vi "uc480_SimpleLive.vi"() -> ()   [LabVIEW 2018]
uses:
  System.Windows.Forms
  C:/Program Files/National Instruments/LabVIEW 2018/uc480DotNet.dll
  Program Files/National Instruments/LabVIEW 2018/uc480DotNet.dll
panel:
  in  "Zoom":u16(ring)=1 items=["4X"=4, "2X"=2, "1X"=1]
  in  "PictureBox":refnum<k24>(container)
  out "Serial Number 2":string
  out "Height 2":i32=8
  out "Width 2":i32=8
  out "Bits/Pixel 2":i32=8
  in  "Camera ID":i32
  out "Serial Number":string
  out "Height":i32=8
  out "Width":i32=8
  out "Bits/Pixel":i32=8
  in  "Pixelclock":i32(slide)=33 min=5 max=30 step=1 scale=5.0..30.0
  in  "Framerate":dbl(slide)=33.21525 min=2.938631097475863 max=10.003070942779434 step=0.008308198457458001 scale=2.938631097475863..10.003070942779434 scale format="%#.3g"
  in  "Exposure":dbl(slide)=33.21525 min=0.11904999999999999 max=99.92214999999999 step=0.0831 scale=0.11904999999999999..99.92214999999999 scale format="%#.3g"
  out "Error Out":errorcluster caption="error"
  in  "Load Parameter":bool
  in  "Exit Camera":bool
  in  "Stop Live":bool
  in  "Start Live":bool
  in  "Init Camera":bool
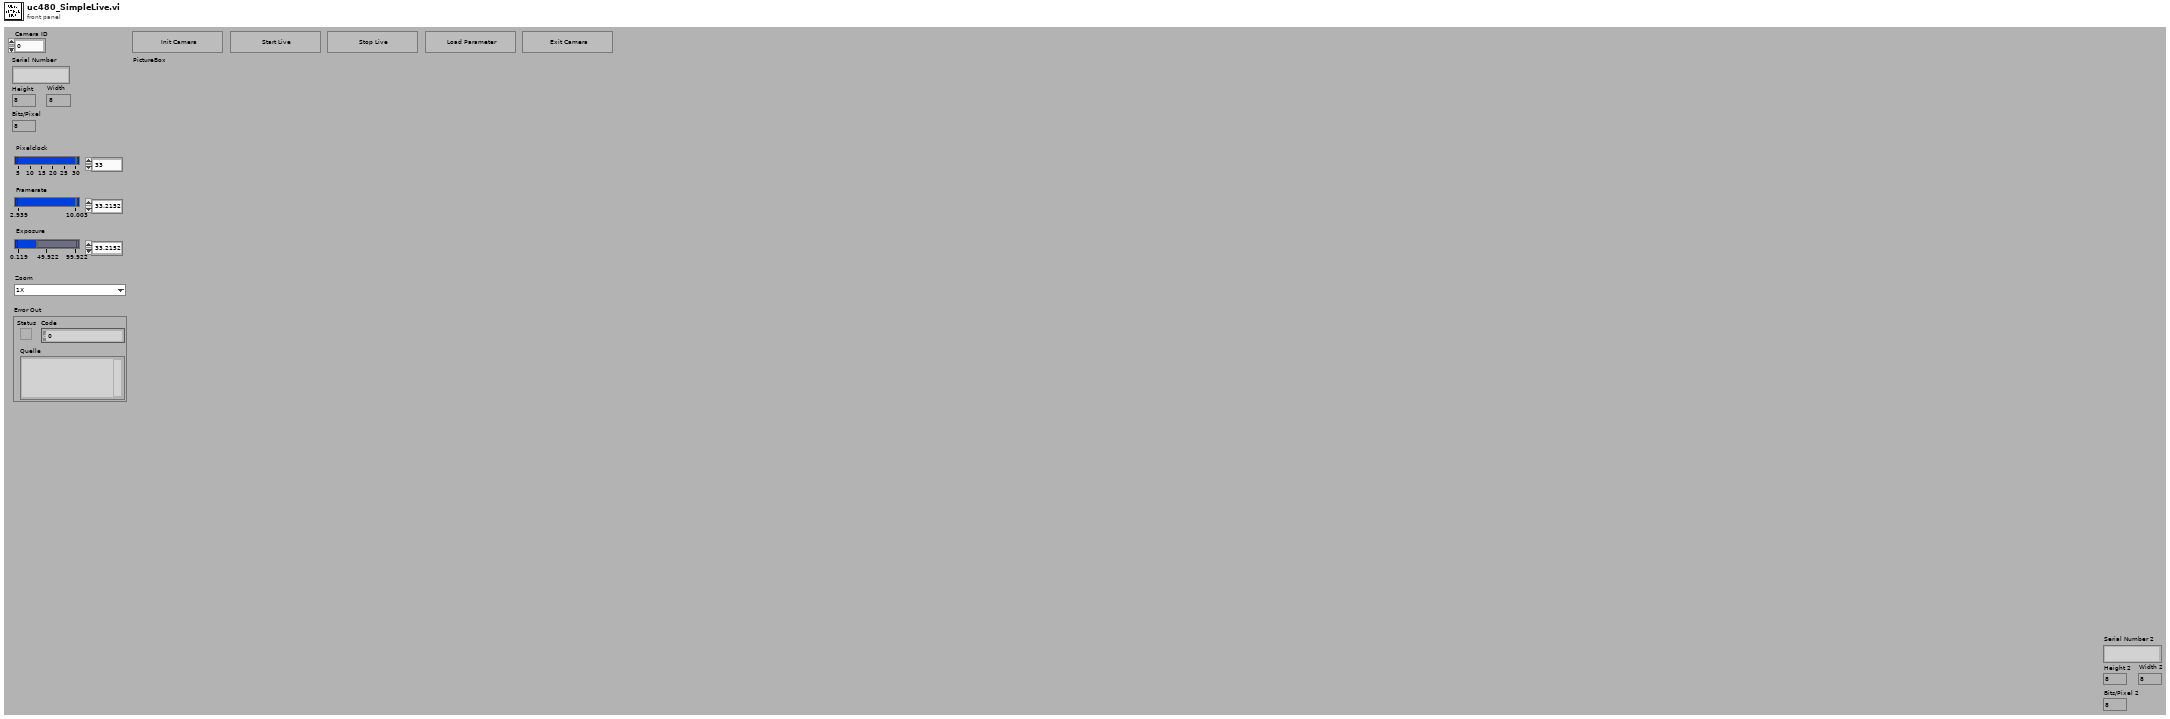
[diagram p1: front panel]
types:
  T1 = enum8{"Enabled", "Disabled", "Disabled and Grayed Out"}
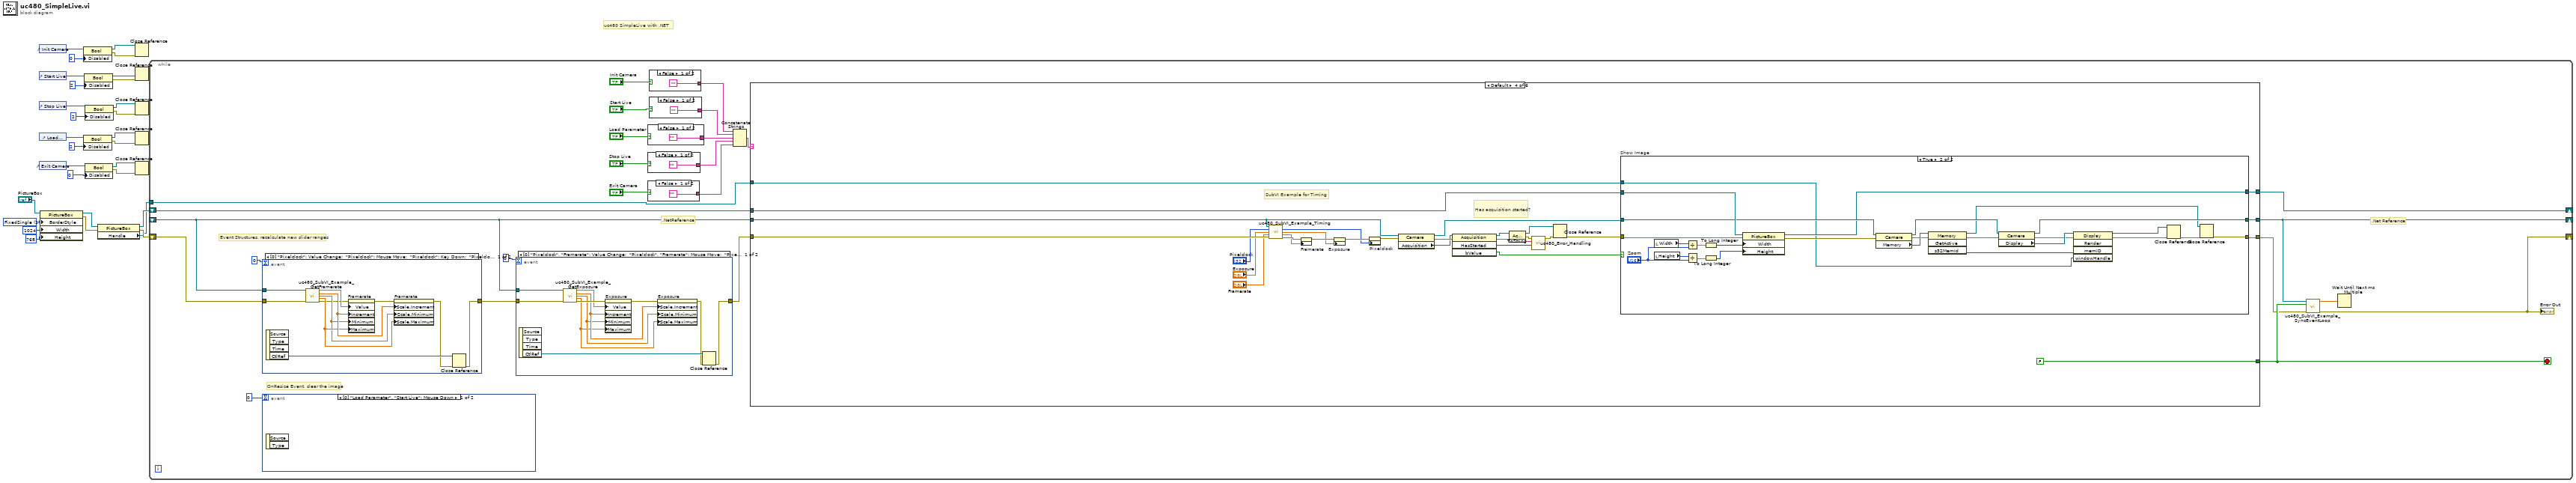
[diagram p0: block diagram]
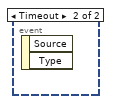
[diagram p2: hidden frame]
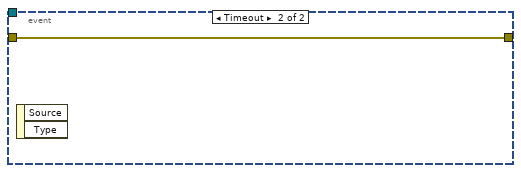
[diagram p3: hidden frame]
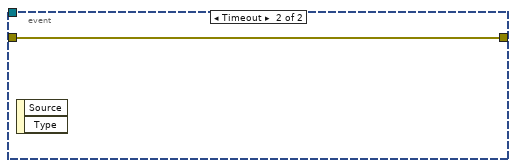
[diagram p4: hidden frame]
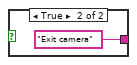
[diagram p5: hidden frame]
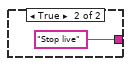
[diagram p6: hidden frame]
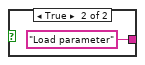
[diagram p7: hidden frame]
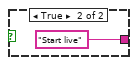
[diagram p8: hidden frame]
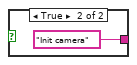
[diagram p9: hidden frame]
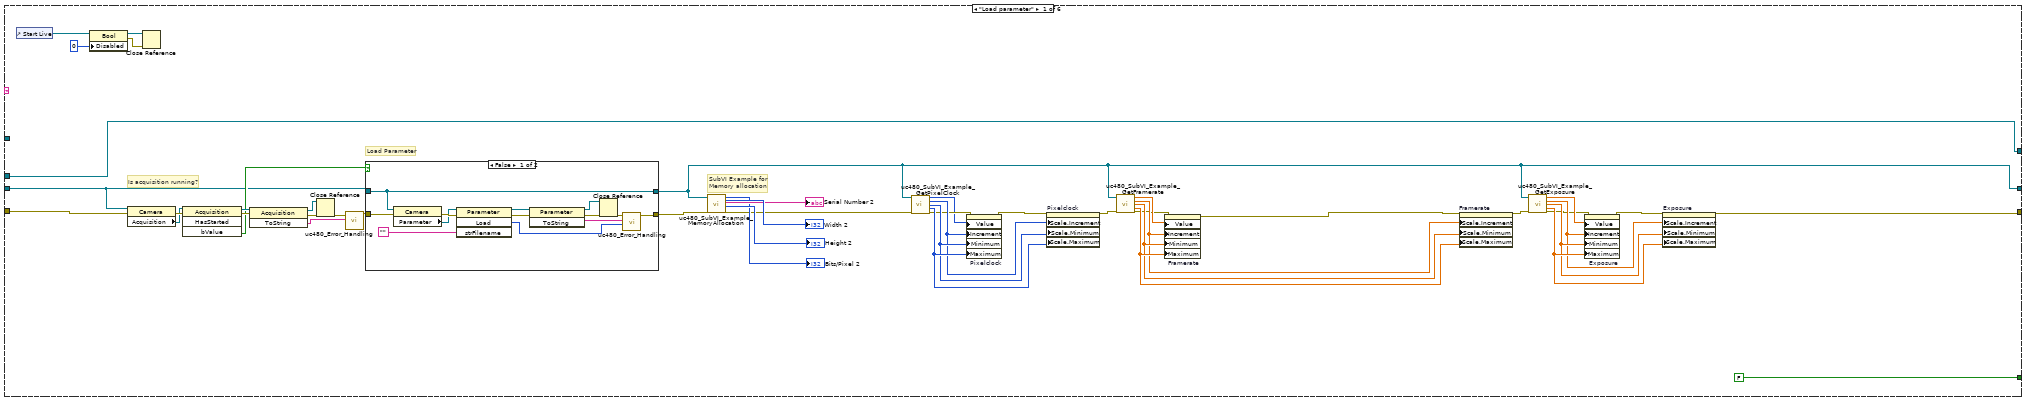
[diagram p10: hidden frame]
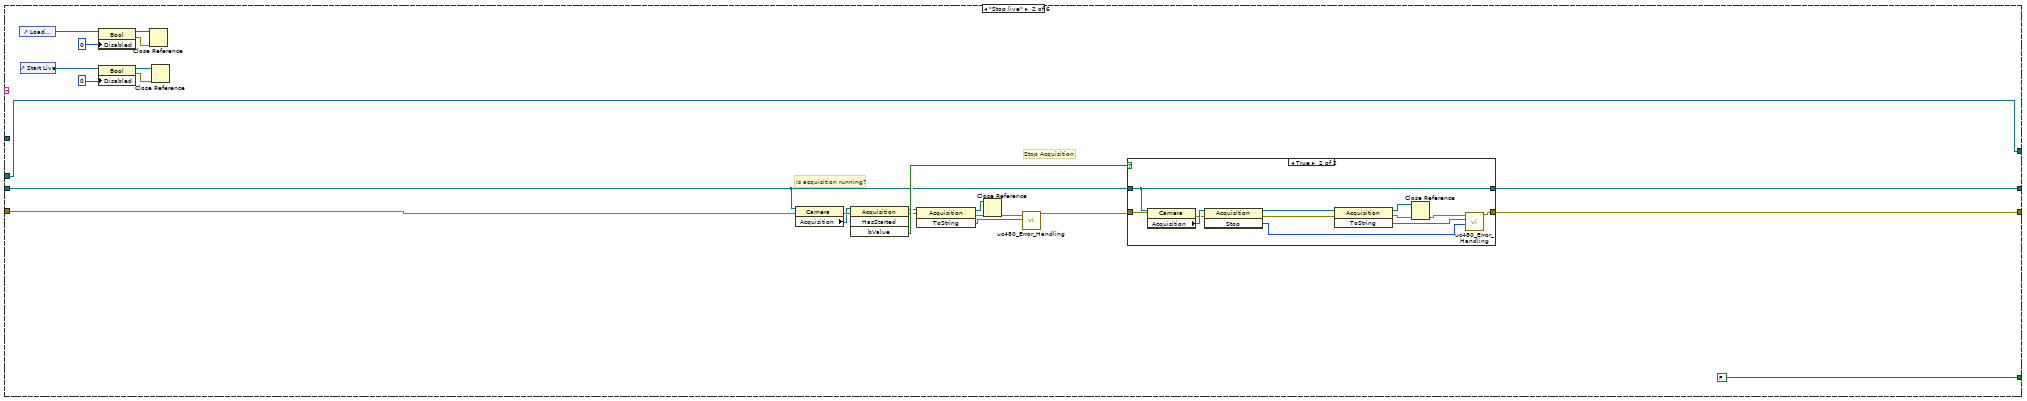
[diagram p12: hidden frame]
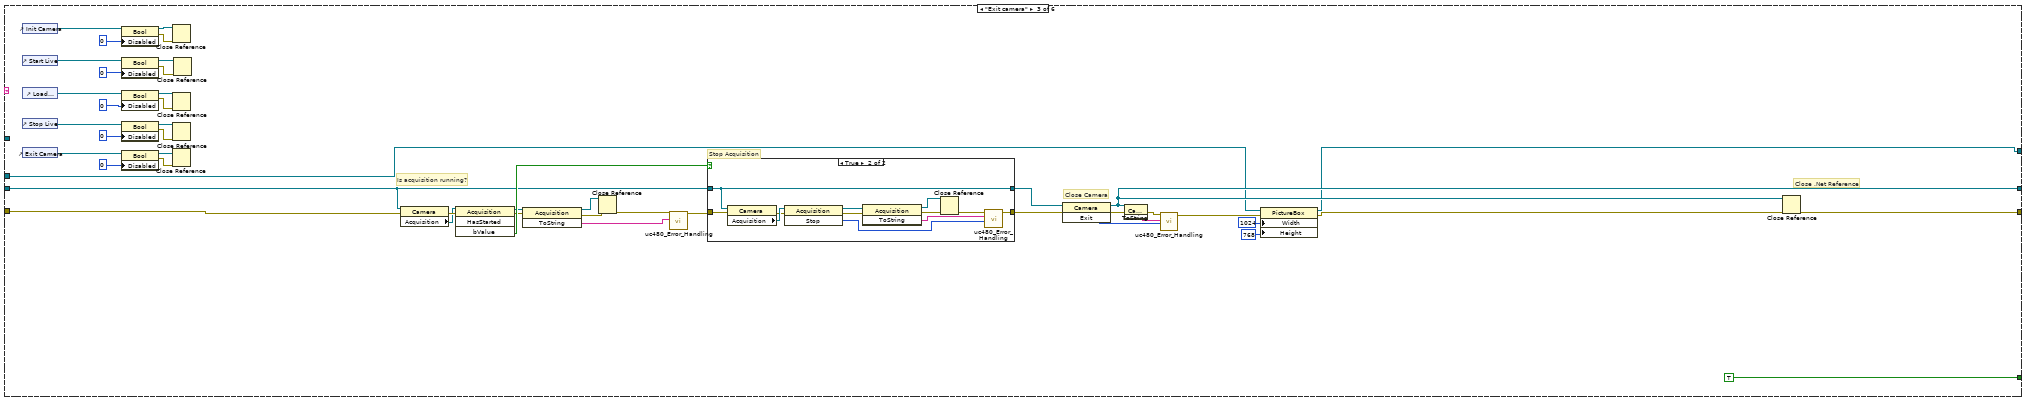
[diagram p14: hidden frame]
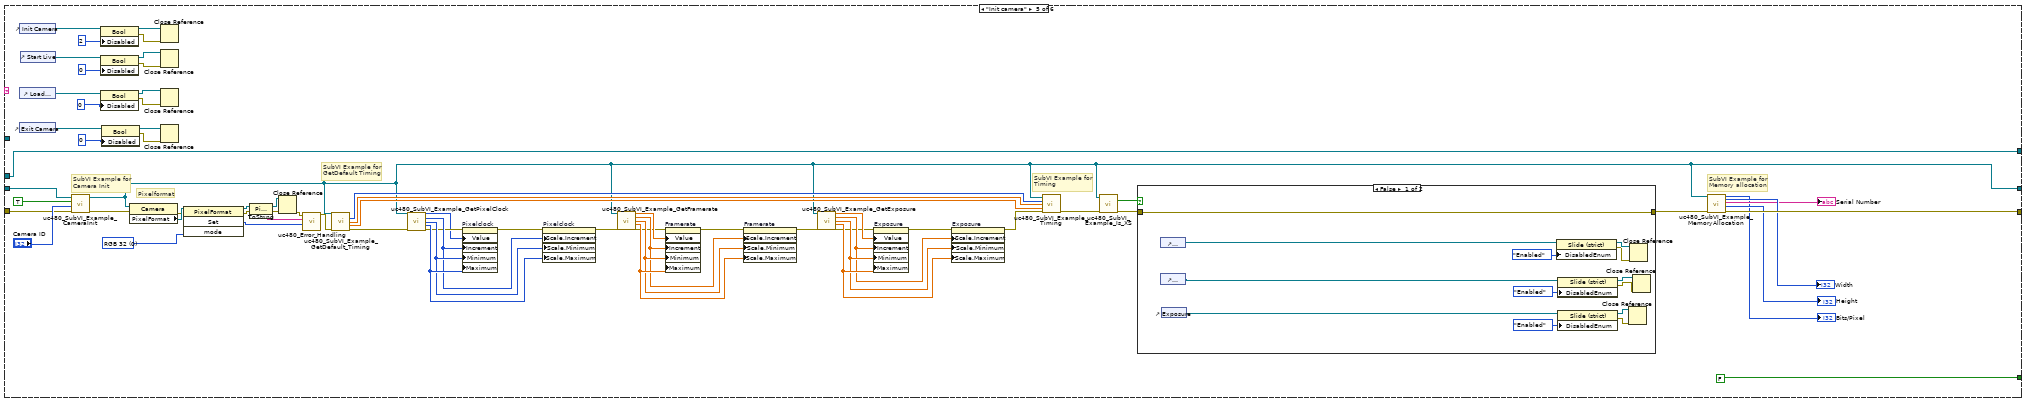
[diagram p17: hidden frame]
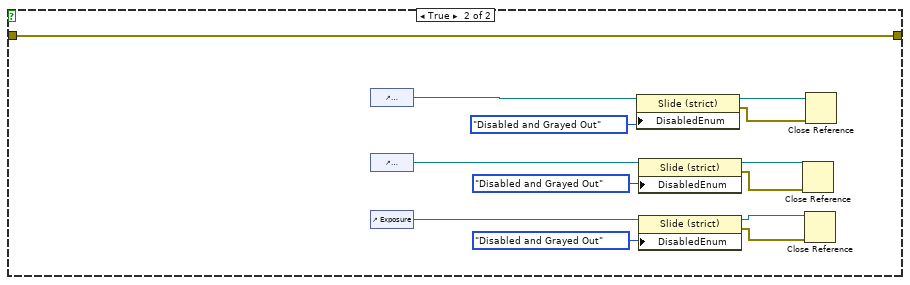
[diagram p18: hidden frame]
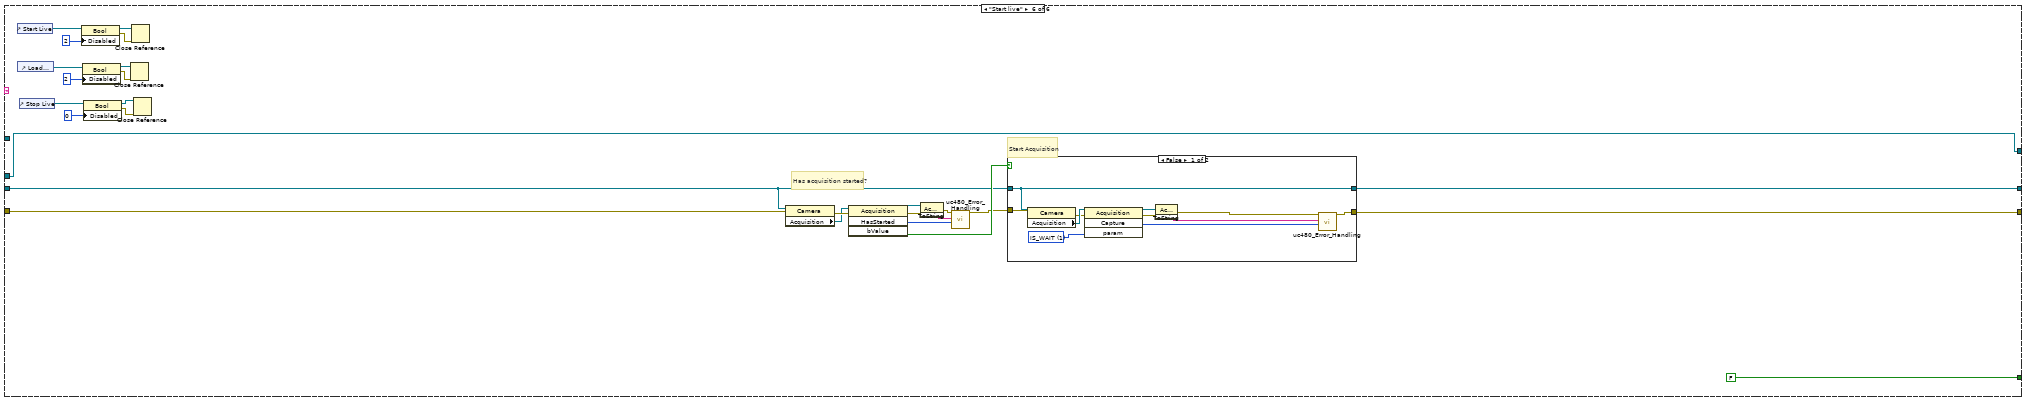
[diagram p19: hidden frame]
diagram:
  w18 = 1 items=["None", "FixedSingle", "Fixed3D"] ("BorderStyle")
  # "uc480 SimpleLive with .NET"
  n1 = control-ref of="Init Camera"() -> (w29:refnum<vi>)
  n2 = control-ref of="Start Live"() -> (w26:refnum<vi>)
  n3 = control-ref of="Stop Live"() -> (w20:refnum<vi>)
  n4 = control-ref of="Load Parameter"() -> (w21:refnum<vi>)
  n5 = control-ref of="Exit Camera"() -> (w22:refnum<vi>)
  n6 = property class="PictureBox"(reference="PictureBox", "BorderStyle"=w18, "Width"=1024, "Height"=768) -> (reference out=w4:refnum<k24>, error out=w5:errorcluster)  [unwired: 1 in]
  n7 = property class="Bool"(reference=w29, "Disabled"=u8 0 ("Deaktiviert")) -> (reference out=w15:refnum<vi>, error out=w14:errorcluster)  [unwired: 1 in]
  n8 = property class="Bool"(reference=w21, "Disabled"=u8 2 ("Deaktiviert")) -> (reference out=w9:refnum<vi>, error out=w8:errorcluster)  [unwired: 1 in]
  n9 = property class="Bool"(reference=w26, "Disabled"=u8 2 ("Deaktiviert")) -> (reference out=w13:refnum<vi>, error out=w12:errorcluster)  [unwired: 1 in]
  n10 = property class="Bool"(reference=w22, "Disabled"=u8 0 ("Deaktiviert")) -> (reference out=w7:refnum<vi>, error out=w6:errorcluster)  [unwired: 1 in]
  n11 = property class="Bool"(reference=w20, "Disabled"=u8 2 ("Deaktiviert")) -> (reference out=w11:refnum<vi>, error out=w10:errorcluster)  [unwired: 1 in]
  n12 = property class="PictureBox"(reference=w4, error in=w5) -> (reference out=w3:refnum<k24>, error out=w2:errorcluster, "Handle"=w1:refnum<k24>)
  n13 = Close Reference(reference=w15, error in (no error)=w14) -> ()  [unwired: 1 out]
  n14 = Close Reference(reference=w13, error in (no error)=w12) -> ()  [unwired: 1 out]
  n15 = Close Reference(reference=w11, error in (no error)=w10) -> ()  [unwired: 1 out]
  n16 = Close Reference(reference=w9, error in (no error)=w8) -> ()  [unwired: 1 out]
  n17 = Close Reference(reference=w7, error in (no error)=w6) -> ()  [unwired: 1 out]
  n18 = while {
    shift-right: [w34] -> _
    shift-left: w2 -> [w40]
    shift-right: [w37] -> _
    shift-left: _ -> [w30]
    shift-right: [w32] -> _
    shift-left: w3 -> [w33]
    tunnel: w1 -> [w31]
    stop <- w38 stop-if-true
    # "OnResize Event, clear the image"
    # "Event Structures, recalculate new slider ranges"
    # ".NetReference"
    # ".Net Reference"
    n19 = event shown="[0] \"Pixelclock\": Value Change;  \"Pixelclock\": Mouse Move;  \"Pixelclock\": Key Down;  \"Pixelclock\": Mouse Up" {
      selector: _ -> [_ _]
      dyn-events: _ -> [_ _]
      timeout: 0 -> [_ _]
      tunnel: [w56 w67] -> w41
      tunnel: w40 -> [w66 w67]
      tunnel: w30 -> [w65 _]
      event "Pixelclock": Value Change; "Pixelclock": Mouse Move; "Pixelclock": Key Down; "Pixelclock": Mouse Up {
        n20 = event-data() -> ("CtlRef"=w58:refnum<vi>)  [unwired: 1 in, 3 out]
        n21 = call "uc480_SubVI_Example_GetFramerate.vi"(".NET (Reference)"=w65, "Error In"=w66) -> ("Framerate"=w64:dbl, "Inc"=w63:dbl, "Min"=w61:dbl, "Max"=w62:dbl, "error out"=w60:errorcluster)  [unwired: 9 in]
        n22 = property on="Framerate" class="Slide (strict)"(error in=w60, "Value"=w64, "Increment"=w63, "Minimum"=w61, "Maximum"=w62) -> (error out=w59:errorcluster)  [unwired: 1 in, 1 out]
        n23 = property on="Framerate" class="Slide (strict)"(error in=w59, "Scale.Increment"=w63, "Scale.Minimum"=w61, "Scale.Maximum"=w62) -> (error out=w57:errorcluster)  [unwired: 1 in, 1 out]
        n24 = Close Reference(reference=w58, error in (no error)=w57) -> (error out=w56:errorcluster)
      }
      event Timeout {
        n25 = event-data() -> ()  [unwired: 1 in, 2 out]
      }
    }
    n26 = event shown="[0] \"Load Parameter\", \"Start Live\": Mouse Down" {
      selector: _ -> [_ _]
      dyn-events: _ -> [_ _]
      timeout: 0 -> [_ _]
      event "Load Parameter", "Start Live": Mouse Down {
        n27 = event-data() -> ()  [unwired: 1 in, 2 out]
      }
      event Timeout {
        n28 = event-data() -> ()  [unwired: 1 in, 2 out]
      }
    }
    n29 = event shown="[0] \"Pixelclock\", \"Framerate\": Value Change;  \"Pixelclock\", \"Framerate\": Mouse Move;  \"Pixelclock\", \"Framerate\": Key Down;  \"Pixelclock\", \"Framerate\": Mouse Up" {
      selector: _ -> [_ _]
      dyn-events: _ -> [_ _]
      timeout: 0 -> [_ _]
      tunnel: w41 -> [w78 w79]
      tunnel: [w68 w79] -> w43
      tunnel: w30 -> [w77 _]
      event "Pixelclock", "Framerate": Value Change; "Pixelclock", "Framerate": Mouse Move; "Pixelclock", "Framerate": Key Down; "Pixelclock", "Framerate": Mouse Up {
        n30 = event-data() -> ("CtlRef"=w70:refnum<vi>)  [unwired: 1 in, 3 out]
        n31 = call "uc480_SubVI_Example_GetExposure.vi"(".NET (Reference)"=w77, "Error In"=w78) -> ("Exposure"=w74:dbl, "Inc"=w73:dbl, "Min"=w72:dbl, "Max"=w71:dbl, "Error out"=w75:errorcluster)  [unwired: 9 in]
        n32 = property on="Exposure" class="Slide (strict)"(error in=w75, "Value"=w74, "Increment"=w73, "Minimum"=w72, "Maximum"=w71) -> (error out=w76:errorcluster)  [unwired: 1 in, 1 out]
        n33 = property on="Exposure" class="Slide (strict)"(error in=w76, "Scale.Increment"=w73, "Scale.Minimum"=w72, "Scale.Maximum"=w71) -> (error out=w69:errorcluster)  [unwired: 1 in, 1 out]
        n34 = Close Reference(reference=w70, error in (no error)=w69) -> (error out=w68:errorcluster)
      }
      event Timeout {
        n35 = event-data() -> ()  [unwired: 1 in, 2 out]
      }
    }
    n36 = case shown="False" "Exit Camera" {
      tunnel: ["" "Exit camera"] -> w45
      frame False {
      }
      frame True {
      }
    }
    n37 = case shown="False" "Load Parameter" {
      tunnel: ["" "Load parameter"] -> w49
      frame False {
      }
      frame True {
      }
    }
    n38 = case shown="False" "Stop Live" {
      tunnel: ["" "Stop live"] -> w48
      frame False {
      }
      frame True {
      }
    }
    n39 = case shown="False" "Init Camera" {
      tunnel: ["" "Init camera"] -> w53
      frame False {
      }
      frame True {
      }
    }
    n40 = case shown="False" "Start Live" {
      tunnel: ["" "Start live"] -> w52
      frame False {
      }
      frame True {
      }
    }
    n41 = Concatenate Strings(w53, w52, w49, w48, w45) -> (w51:string)
    n42 = case shown="Default" w51 {
      tunnel: w30 -> [w126 w166 w220 w262 w369 w420]
      tunnel: w43 -> [w129 w167 w221 w272 w368 w421]
      tunnel: [w96 w165 w229 w271 w325 w419] -> w37
      tunnel: [w97 w164 w230 w270 w364 w417] -> w36
      tunnel: [FALSE FALSE TRUE FALSE FALSE FALSE] -> w38
      tunnel: w33 -> [w95 w158 w200 w254 w320 w410]
      tunnel: [w95 w158 w199 w253 w320 w410] -> w32
      tunnel: w31 -> [_ _ _ w250 _ _]
      frame "Load parameter" {
        # "SubVI Example for \nMemory allocation"
        # "Is acquisition running?"
        # "Load Parameter"
        n43 = control-ref of="Start Live"() -> (w120:refnum<vi>)
        n44 = property class="Bool"(reference=w120, "Disabled"=u8 0 ("Deaktiviert")) -> (reference out=w94:refnum<vi>, error out=w93:errorcluster)  [unwired: 1 in]
        n45 = property class="Camera"(reference=w126, error in=w129) -> (error out=w134:errorcluster, "Acquisition"=w133:refnum<k24>)  [unwired: 1 out]
        n46 = Close Reference(reference=w94, error in (no error)=w93) -> ()  [unwired: 1 out]
        n47 = invoke class="Acquisition" method="HasStarted"(reference=w133, error in=w134) -> (reference out=w130:refnum<k24>, error out=w132:errorcluster, "bValue"=w128:bool)  [unwired: 2 in, 1 out]
        n48 = invoke class="Acquisition" method="ToString"(reference=w130, error in=w132) -> (reference out=w92:refnum<k24>, error out=w91:errorcluster, "ToString"=w131:string)  [unwired: 1 in]
        n49 = Close Reference(reference=w92, error in (no error)=w91) -> (error out=w90:errorcluster)
        n50 = call "uc480_Error_Handling.vi"("Error String"=w131, "Error In"=w90) -> ("Error Out"=w127:errorcluster)  [unwired: 9 in]
        n51 = case shown="False" w128 {
          tunnel: w127 -> [w142 w149]
          tunnel: w126 -> [w140 w150]
          tunnel: [w141 w149] -> w121
          tunnel: [w140 w150] -> w96
          frame False {
            n52 = property class="Camera"(reference=w140, error in=w142) -> (error out=w144:errorcluster, "Parameter"=w143:refnum<k24>)  [unwired: 1 out]
            n53 = invoke class="Parameter" method="Load"(reference=w143, error in=w144, "strFilename"="") -> (reference out=w146:refnum<k24>, error out=w147:errorcluster, "Load"=w139:i32)  [unwired: 1 in, 1 out]
            n54 = invoke class="Parameter" method="ToString"(reference=w146, error in=w147) -> (reference out=w136:refnum<k24>, error out=w138:errorcluster, "ToString"=w148:string)  [unwired: 1 in]
            n55 = Close Reference(reference=w136, error in (no error)=w138) -> (error out=w137:errorcluster)
            n56 = call "uc480_Error_Handling.vi"("Error Code"=w139, "Error String"=w148, "Error In"=w137) -> ("Error Out"=w141:errorcluster)  [unwired: 8 in]
          }
          frame True {
          }
        }
        n57 = call "uc480_SubVI_Example_MemoryAllocation.vi"(".NET (Reference)"=w96, "Error In"=w121) -> ("Bits/Pixel 2"=→"Bits/Pixel 2":i32, "Width"=→"Width 2":i32, "Serial Number"=→"Serial Number 2":string, "Height"=→"Height 2":i32, "Error Out"=w98:errorcluster)  [unwired: 13 in]
        n58 = call "uc480_SubVI_Example_GetPixelClock.vi"(".NET (Reference)"=w96, "Error In"=w98) -> ("Pixel Clock"=w99:i32, "Inc"=w101:i32, "Min"=w102:i32, "Max"=w103:i32, "error out"=w100:errorcluster)  [unwired: 9 in]
        n59 = property on="Pixelclock" class="Slide (strict)"(error in=w100, "Value"=w99, "Increment"=w101, "Minimum"=w102, "Maximum"=w103) -> (error out=w104:errorcluster)  [unwired: 1 in, 1 out]
        n60 = property on="Pixelclock" class="Slide (strict)"(error in=w104, "Scale.Increment"=w101, "Scale.Minimum"=w102, "Scale.Maximum"=w103) -> (error out=w105:errorcluster)  [unwired: 1 in, 1 out]
        n61 = call "uc480_SubVI_Example_GetFramerate.vi"(".NET (Reference)"=w96, "Error In"=w105) -> ("Framerate"=w108:dbl, "Inc"=w109:dbl, "Min"=w110:dbl, "Max"=w111:dbl, "error out"=w107:errorcluster)  [unwired: 9 in]
        n62 = property on="Framerate" class="Slide (strict)"(error in=w107, "Value"=w108, "Increment"=w109, "Minimum"=w110, "Maximum"=w111) -> (error out=w106:errorcluster)  [unwired: 1 in, 1 out]
        n63 = property on="Framerate" class="Slide (strict)"(error in=w106, "Scale.Increment"=w109, "Scale.Minimum"=w110, "Scale.Maximum"=w111) -> (error out=w112:errorcluster)  [unwired: 1 in, 1 out]
        n64 = call "uc480_SubVI_Example_GetExposure.vi"(".NET (Reference)"=w96, "Error In"=w112) -> ("Exposure"=w115:dbl, "Inc"=w116:dbl, "Min"=w117:dbl, "Max"=w118:dbl, "Error out"=w113:errorcluster)  [unwired: 9 in]
        n65 = property on="Exposure" class="Slide (strict)"(error in=w113, "Value"=w115, "Increment"=w116, "Minimum"=w117, "Maximum"=w118) -> (error out=w114:errorcluster)  [unwired: 1 in, 1 out]
        n66 = property on="Exposure" class="Slide (strict)"(error in=w114, "Scale.Increment"=w116, "Scale.Minimum"=w117, "Scale.Maximum"=w118) -> (error out=w97:errorcluster)  [unwired: 1 in, 1 out]
      }
      frame "Stop live" {
        # "Is acquisition running?"
        # "Stop Acquisition"
        n67 = control-ref of="Load Parameter"() -> (w162:refnum<vi>)
        n68 = control-ref of="Start Live"() -> (w159:refnum<vi>)
        n69 = property class="Bool"(reference=w162, "Disabled"=u8 0 ("Deaktiviert")) -> (reference out=w157:refnum<vi>, error out=w156:errorcluster)  [unwired: 1 in]
        n70 = property class="Bool"(reference=w159, "Disabled"=u8 0 ("Deaktiviert")) -> (reference out=w155:refnum<vi>, error out=w154:errorcluster)  [unwired: 1 in]
        n71 = Close Reference(reference=w157, error in (no error)=w156) -> ()  [unwired: 1 out]
        n72 = Close Reference(reference=w155, error in (no error)=w154) -> ()  [unwired: 1 out]
        n73 = property class="Camera"(reference=w166, error in=w167) -> (error out=w174:errorcluster, "Acquisition"=w173:refnum<k24>)  [unwired: 1 out]
        n74 = invoke class="Acquisition" method="HasStarted"(reference=w173, error in=w174) -> (reference out=w168:refnum<k24>, error out=w170:errorcluster, "bValue"=w172:bool)  [unwired: 2 in, 1 out]
        n75 = invoke class="Acquisition" method="ToString"(reference=w168, error in=w170) -> (reference out=w151:refnum<k24>, error out=w153:errorcluster, "ToString"=w169:string)  [unwired: 1 in]
        n76 = Close Reference(reference=w151, error in (no error)=w153) -> (error out=w152:errorcluster)
        n77 = call "uc480_Error_Handling.vi"("Error String"=w169, "Error In"=w152) -> ("Error Out"=w171:errorcluster)  [unwired: 9 in]
        n78 = case shown="True" w172 {
          tunnel: [w176 w187] -> w164
          tunnel: w171 -> [w176 w188]
          tunnel: w166 -> [w175 w180]
          tunnel: [w175 w180] -> w165
          frame False {
          }
          frame True {
            n79 = property class="Camera"(reference=w180, error in=w188) -> (error out=w184:errorcluster, "Acquisition"=w185:refnum<k24>)  [unwired: 1 out]
            n80 = invoke class="Acquisition" method="Stop"(reference=w185, error in=w184) -> (reference out=w182:refnum<k24>, error out=w183:errorcluster, "Stop"=w181:i32)  [unwired: 1 in]
            n81 = invoke class="Acquisition" method="ToString"(reference=w182, error in=w183) -> (reference out=w177:refnum<k24>, error out=w179:errorcluster, "ToString"=w186:string)  [unwired: 1 in]
            n82 = Close Reference(reference=w177, error in (no error)=w179) -> (error out=w178:errorcluster)
            n83 = call "uc480_Error_Handling.vi"("Error Code"=w181, "Error String"=w186, "Error In"=w178) -> ("Error Out"=w187:errorcluster)  [unwired: 8 in]
          }
        }
      }
      frame "Exit camera" {
        # "Close .Net Reference"
        # "Is acquisition running?"
        # "Stop Acquisition"
        # "Close Camera"
        n84 = control-ref of="Init Camera"() -> (w212:refnum<vi>)
        n85 = control-ref of="Start Live"() -> (w211:refnum<vi>)
        n86 = control-ref of="Load Parameter"() -> (w210:refnum<vi>)
        n87 = control-ref of="Stop Live"() -> (w209:refnum<vi>)
        n88 = control-ref of="Exit Camera"() -> (w208:refnum<vi>)
        n89 = property class="Bool"(reference=w212, "Disabled"=u8 0 ("Deaktiviert")) -> (reference out=w190:refnum<vi>, error out=w189:errorcluster)  [unwired: 1 in]
        n90 = property class="Bool"(reference=w211, "Disabled"=u8 0 ("Deaktiviert")) -> (reference out=w192:refnum<vi>, error out=w191:errorcluster)  [unwired: 1 in]
        n91 = property class="Bool"(reference=w210, "Disabled"=u8 0 ("Deaktiviert")) -> (reference out=w194:refnum<vi>, error out=w193:errorcluster)  [unwired: 1 in]
        n92 = property class="Bool"(reference=w209, "Disabled"=u8 0 ("Deaktiviert")) -> (reference out=w196:refnum<vi>, error out=w195:errorcluster)  [unwired: 1 in]
        n93 = property class="Bool"(reference=w208, "Disabled"=u8 0 ("Deaktiviert")) -> (reference out=w198:refnum<vi>, error out=w197:errorcluster)  [unwired: 1 in]
        n94 = Close Reference(reference=w190, error in (no error)=w189) -> ()  [unwired: 1 out]
        n95 = Close Reference(reference=w198, error in (no error)=w197) -> ()  [unwired: 1 out]
        n96 = Close Reference(reference=w194, error in (no error)=w193) -> ()  [unwired: 1 out]
        n97 = Close Reference(reference=w196, error in (no error)=w195) -> ()  [unwired: 1 out]
        n98 = Close Reference(reference=w192, error in (no error)=w191) -> ()  [unwired: 1 out]
        n99 = property class="Camera"(reference=w220, error in=w221) -> (error out=w228:errorcluster, "Acquisition"=w227:refnum<k24>)  [unwired: 1 out]
        n100 = invoke class="Acquisition" method="HasStarted"(reference=w227, error in=w228) -> (reference out=w222:refnum<k24>, error out=w224:errorcluster, "bValue"=w226:bool)  [unwired: 2 in, 1 out]
        n101 = invoke class="Acquisition" method="ToString"(reference=w222, error in=w224) -> (reference out=w205:refnum<k24>, error out=w207:errorcluster, "ToString"=w223:string)  [unwired: 1 in]
        n102 = Close Reference ("Close Referenz")(reference=w205, error in (no error)=w207) -> (error out=w206:errorcluster)
        n103 = call "uc480_Error_Handling.vi"("Error String"=w223, "Error In"=w206) -> ("Error Out"=w225:errorcluster)  [unwired: 9 in]
        n104 = case shown="True" w226 {
          tunnel: [w237 w248] -> w218
          tunnel: w225 -> [w237 w249]
          tunnel: w220 -> [w236 w241]
          tunnel: [w236 w241] -> w219
          frame False {
          }
          frame True {
            n105 = property class="Camera"(reference=w241, error in=w249) -> (error out=w245:errorcluster, "Acquisition"=w246:refnum<k24>)  [unwired: 1 out]
            n106 = invoke class="Acquisition" method="Stop"(reference=w246, error in=w245) -> (reference out=w243:refnum<k24>, error out=w244:errorcluster, "Stop"=w242:i32)  [unwired: 1 in]
            n107 = invoke class="Acquisition" method="ToString"(reference=w243, error in=w244) -> (reference out=w238:refnum<k24>, error out=w240:errorcluster, "ToString"=w247:string)  [unwired: 1 in]
            n108 = Close Reference ("Close Referenz")(reference=w238, error in (no error)=w240) -> (error out=w239:errorcluster)
            n109 = call "uc480_Error_Handling.vi"("Error Code"=w242, "Error String"=w247, "Error In"=w239) -> ("Error Out"=w248:errorcluster)  [unwired: 8 in]
          }
        }
        n110 = invoke class="Camera" method="Exit"(reference=w219, error in=w218) -> (reference out=w229:refnum<k24>, error out=w232:errorcluster, "Exit"=w231:i32)  [unwired: 1 in]
        n111 = invoke class="Camera" method="ToString"(reference=w229, error in=w232) -> (error out=w233:errorcluster, "ToString"=w234:string)  [unwired: 1 in, 1 out]
        n112 = call "uc480_Error_Handling.vi"("Error Code"=w231, "Error String"=w234, "Error In"=w233) -> ("Error Out"=w204:errorcluster)  [unwired: 8 in]
        n113 = property class="PictureBox"(reference=w200, error in=w204, "Width"=1024, "Height"=768) -> (reference out=w199:refnum<k24>, error out=w203:errorcluster)
        n114 = Close Reference ("Close Referenz")(reference=w229, error in (no error)=w203) -> (error out=w230:errorcluster)
      }
      frame Default {
        # "SubVI Example for Timing"
        # "Has acquisition started?"
        n115 = call "uc480_SubVI_Example_Timing.vi"(".NET (Reference)"=w262, "Pixelclock"="Pixelclock", "Exposure time"="Exposure", "Framerate"="Framerate", "Error In"=w272) -> ("Pixelclock"=w265:i32, "Exposure time"=w264:dbl, "Framerate"=w263:dbl, "Error Out"=w269:errorcluster)  [unwired: 7 in]
        n116 = property on="Framerate" class="Schieber (strikt)"(error in=w269, "Scale.RngStart"=w263) -> (error out=w268:errorcluster)  [unwired: 1 in, 1 out]
        n117 = property on="Exposure" class="Schieber (strikt)"(error in=w268, "Scale.RngStart"=w264) -> (error out=w267:errorcluster)  [unwired: 1 in, 1 out]
        n118 = property on="Pixelclock" class="Schieber (strikt)"(error in=w267, "Scale.RngStart"=w265) -> (error out=w266:errorcluster)  [unwired: 1 in, 1 out]
        n119 = property class="Camera"(reference=w262, error in=w266) -> (reference out=w255:refnum<k24>, error out=w278:errorcluster, "Acquisition"=w277:refnum<k24>)
        n120 = invoke class="Acquisition" method="HasStarted"(reference=w277, error in=w278) -> (reference out=w252:refnum<k24>, error out=w274:errorcluster, "HasStarted"=w273:i32, "bValue"=w251:bool)  [unwired: 2 in]
        n121 = invoke class="Acquisition" method="ToString"(reference=w252, error in=w274) -> (reference out=w256:refnum<k24>, error out=w276:errorcluster, "ToString"=w275:string)  [unwired: 1 in]
        n122 = call "uc480_Error_Handling.vi"("Error Code"=w273, "Error String"=w275, "Error In"=w276) -> ("Error Out"=w258:errorcluster)  [unwired: 8 in]
        n123 = Close Reference(reference=w256, error in (no error)=w258) -> (error out=w257:errorcluster)
        n124 = case "Show Image" shown="True" w251 {
          tunnel: [w282 w288] -> w270
          tunnel: w257 -> [w282 w299]
          tunnel: w255 -> [w281 w298]
          tunnel: [w281 w303] -> w271
          tunnel: w254 -> [w280 w300]
          tunnel: [w280 w284] -> w253
          tunnel: w250 -> [_ w283]
          frame False {
          }
          frame True {
            n125 = local read "Height"() -> (w296:i32)
            n126 = local read "Width"() -> (w292:i32)
            n127 = Divide(x=w292, y="Zoom") -> (x/y=w294:dbl)
            n128 = Divide(x=w296, y="Zoom") -> (x/y=w297:dbl)
            n129 = To Long Integer(number=w294) -> (32bit integer=w293:i32)
            n130 = To Long Integer(number=w297) -> (32bit integer=w295:i32)
            n131 = property class="PictureBox"(reference=w300, error in=w299, "Width"=w293, "Height"=w295) -> (reference out=w284:refnum<k24>, error out=w285:errorcluster)
            n132 = property class="Camera"(reference=w298, error in=w285) -> (reference out=w304:refnum<k24>, error out=w307:errorcluster, "Memory"=w308:refnum<k24>)
            n133 = invoke class="Memory" method="GetActive"(reference=w308, error in=w307) -> (reference out=w286:refnum<k24>, error out=w287:errorcluster, "s32MemId"=w302:i32)  [unwired: 2 in, 1 out]
            n134 = property class="Camera"(reference=w304, error in=w287) -> (reference out=w303:refnum<k24>, error out=w301:errorcluster, "Display"=w306:refnum<k24>)
            n135 = invoke class="Display" method="Render"(reference=w306, error in=w301, "memID"=w302, "windowHandle"=w283) -> (reference out=w305:refnum<k24>, error out=w290:errorcluster)  [unwired: 1 in, 3 out]
            n136 = Close Reference(reference=w305, error in (no error)=w290) -> (error out=w289:errorcluster)
            n137 = Close Reference(reference=w286, error in (no error)=w289) -> (error out=w288:errorcluster)
          }
        }
      }
      frame "Init camera" {
        w377 = 0 items=["RGB 32"=0, "RGB 24"=1, "Y8 Monochrom"=6] ("Mode")
        # "SubVI Example for \nGetDefault Timing"
        # "SubVI Example for \nMemory allocation"
        # "SubVI Example for \nTiming"
        # "SubVI Example for \nCamera Init"
        # "Pixelformat"
        n138 = control-ref of="Init Camera"() -> (w332:refnum<vi>)
        n139 = control-ref of="Load Parameter"() -> (w328:refnum<vi>)
        n140 = control-ref of="Exit Camera"() -> (w326:refnum<vi>)
        n141 = control-ref of="Start Live"() -> (w330:refnum<vi>)
        n142 = call "uc480_SubVI_Example_CameraInit.vi"("Error In"=w368, "Camera ID"="Camera ID", "Init Camera Flag"=TRUE, ".NET (Reference)"=w369) -> ("Error Out"=w374:errorcluster, ".NET (Reference)"=w325:refnum<k24>)  [unwired: 6 in]
        n143 = property class="Bool"(reference=w328, "Disabled"=u8 0 ("Deaktiviert")) -> (reference out=w315:refnum<vi>, error out=w314:errorcluster)  [unwired: 1 in]
        n144 = property class="Bool"(reference=w332, "Disabled"=u8 2 ("Deaktiviert")) -> (reference out=w319:refnum<vi>, error out=w318:errorcluster)  [unwired: 1 in]
        n145 = property class="Bool"(reference=w330, "Disabled"=u8 0 ("Deaktiviert")) -> (reference out=w317:refnum<vi>, error out=w316:errorcluster)  [unwired: 1 in]
        n146 = property class="Bool"(reference=w326, "Disabled"=u8 0 ("Deaktiviert")) -> (reference out=w313:refnum<vi>, error out=w312:errorcluster)  [unwired: 1 in]
        n147 = property on="Property Node" class="Camera"(reference=w325, error in=w374) -> (error out=w375:errorcluster, "PixelFormat"=w376:refnum<k24>)  [unwired: 1 out]
        n148 = Close Reference(reference=w319, error in (no error)=w318) -> ()  [unwired: 1 out]
        n149 = Close Reference(reference=w317, error in (no error)=w316) -> ()  [unwired: 1 out]
        n150 = Close Reference(reference=w315, error in (no error)=w314) -> ()  [unwired: 1 out]
        n151 = Close Reference(reference=w313, error in (no error)=w312) -> ()  [unwired: 1 out]
        n152 = invoke class="PixelFormat" method="Set"(reference=w376, error in=w375, "mode"=w377) -> (reference out=w372:refnum<k24>, error out=w365:errorcluster, "Set"=w371:i32)  [unwired: 1 in, 1 out]
        n153 = invoke class="PixelFormat" method="ToString"(reference=w372, error in=w365) -> (reference out=w309:refnum<k24>, error out=w311:errorcluster, "ToString"=w373:string)  [unwired: 1 in]
        n154 = Close Reference(reference=w309, error in (no error)=w311) -> (error out=w310:errorcluster)
        n155 = call "uc480_Error_Handling.vi"("Error Code"=w371, "Error String"=w373, "Error In"=w310) -> ("Error Out"=w339:errorcluster)  [unwired: 8 in]
        n156 = call "uc480_SubVI_Example_GetDefault_Timing.vi"(".NET (Reference)"=w325, "Error In"=w339) -> ("Pixelclock"=w338:i32, "Exposure time"=w337:dbl, "Framerate"=w336:dbl, "Error Out"=w335:errorcluster)  [unwired: 10 in]
        n157 = call "uc480_SubVI_Example_GetPixelClock.vi"(".NET (Reference)"=w325, "Error In"=w335) -> ("Pixel Clock"=w340:i32, "Inc"=w342:i32, "Min"=w343:i32, "Max"=w344:i32, "error out"=w341:errorcluster)  [unwired: 9 in]
        n158 = property on="Pixelclock" class="Slide (strict)"(error in=w341, "Value"=w340, "Increment"=w342, "Minimum"=w343, "Maximum"=w344) -> (error out=w345:errorcluster)  [unwired: 1 in, 1 out]
        n159 = property on="Pixelclock" class="Slide (strict)"(error in=w345, "Scale.Increment"=w342, "Scale.Minimum"=w343, "Scale.Maximum"=w344) -> (error out=w346:errorcluster)  [unwired: 1 in, 1 out]
        n160 = call "uc480_SubVI_Example_GetFramerate.vi"(".NET (Reference)"=w325, "Error In"=w346) -> ("Framerate"=w349:dbl, "Inc"=w350:dbl, "Min"=w351:dbl, "Max"=w352:dbl, "error out"=w348:errorcluster)  [unwired: 9 in]
        n161 = property on="Framerate" class="Slide (strict)"(error in=w348, "Value"=w349, "Increment"=w350, "Minimum"=w351, "Maximum"=w352) -> (error out=w347:errorcluster)  [unwired: 1 in, 1 out]
        n162 = property on="Framerate" class="Slide (strict)"(error in=w347, "Scale.Increment"=w350, "Scale.Minimum"=w351, "Scale.Maximum"=w352) -> (error out=w353:errorcluster)  [unwired: 1 in, 1 out]
        n163 = call "uc480_SubVI_Example_GetExposure.vi"(".NET (Reference)"=w325, "Error In"=w353) -> ("Exposure"=w356:dbl, "Inc"=w357:dbl, "Min"=w358:dbl, "Max"=w359:dbl, "Error out"=w354:errorcluster)  [unwired: 9 in]
        n164 = property on="Exposure" class="Slide (strict)"(error in=w354, "Value"=w356, "Increment"=w357, "Minimum"=w358, "Maximum"=w359) -> (error out=w355:errorcluster)  [unwired: 1 in, 1 out]
        n165 = property on="Exposure" class="Slide (strict)"(error in=w355, "Scale.Increment"=w357, "Scale.Minimum"=w358, "Scale.Maximum"=w359) -> (error out=w334:errorcluster)  [unwired: 1 in, 1 out]
        n166 = call "uc480_SubVI_Example_Timing.vi"(".NET (Reference)"=w325, "Pixelclock"=w338, "Exposure time"=w337, "Framerate"=w336, "Error In"=w334) -> ("Error Out"=w324:errorcluster)  [unwired: 7 in, 3 out]
        n167 = call "uc480_SubVI_Example_Is_XS.vi"("Error In"=w324, ".NET (Reference)"=w325) -> ("Error Out"=w321:errorcluster, "IsXS"=w323:bool)  [unwired: 7 in, 1 out]
        n168 = case shown="False" w323 {
          tunnel: w321 -> [w390 w403]
          tunnel: [w390 w403] -> w322
          frame False {
            n169 = control-ref of="Pixelclock"() -> (w386:refnum<vi>)
            n170 = control-ref of="Framerate"() -> (w385:refnum<vi>)
            n171 = control-ref of="Exposure"() -> (w384:refnum<vi>)
            n172 = property class="Slide (strict)"(reference=w386, "DisabledEnum"=T1."Enabled" ("Disabled")) -> (reference out=w383:refnum<vi>, error out=w382:errorcluster)  [unwired: 1 in]
            n173 = property class="Slide (strict)"(reference=w385, "DisabledEnum"=T1."Enabled" ("Disabled")) -> (reference out=w381:refnum<vi>, error out=w380:errorcluster)  [unwired: 1 in]
            n174 = property class="Slide (strict)"(reference=w384, "DisabledEnum"=T1."Enabled" ("Disabled")) -> (reference out=w379:refnum<vi>, error out=w378:errorcluster)  [unwired: 1 in]
            n175 = Close Reference(reference=w379, error in (no error)=w378) -> ()  [unwired: 1 out]
            n176 = Close Reference(reference=w383, error in (no error)=w382) -> ()  [unwired: 1 out]
            n177 = Close Reference(reference=w381, error in (no error)=w380) -> ()  [unwired: 1 out]
          }
          frame True {
            n178 = control-ref of="Pixelclock"() -> (w402:refnum<vi>)
            n179 = control-ref of="Framerate"() -> (w399:refnum<vi>)
            n180 = control-ref of="Exposure"() -> (w397:refnum<vi>)
            n181 = property class="Slide (strict)"(reference=w402, "DisabledEnum"=T1."Disabled and Grayed Out" ("Disabled")) -> (reference out=w395:refnum<vi>, error out=w396:errorcluster)  [unwired: 1 in]
            n182 = property class="Slide (strict)"(reference=w399, "DisabledEnum"=T1."Disabled and Grayed Out" ("Disabled")) -> (reference out=w394:refnum<vi>, error out=w393:errorcluster)  [unwired: 1 in]
            n183 = property class="Slide (strict)"(reference=w397, "DisabledEnum"=T1."Disabled and Grayed Out" ("Disabled")) -> (reference out=w392:refnum<vi>, error out=w391:errorcluster)  [unwired: 1 in]
            n184 = Close Reference(reference=w394, error in (no error)=w393) -> ()  [unwired: 1 out]
            n185 = Close Reference(reference=w392, error in (no error)=w391) -> ()  [unwired: 1 out]
            n186 = Close Reference(reference=w395, error in (no error)=w396) -> ()  [unwired: 1 out]
          }
        }
        n187 = call "uc480_SubVI_Example_MemoryAllocation.vi"(".NET (Reference)"=w325, "Error In"=w322) -> ("Bits/Pixel 2"=→"Bits/Pixel":i32, "Width"=→"Width":i32, "Serial Number"=→"Serial Number":string, "Height"=→"Height":i32, "Error Out"=w364:errorcluster)  [unwired: 13 in]
      }
      frame "Start live" {
        # "Has acquisition started?"
        # "Start Acquisition"
        n188 = control-ref of="Start Live"() -> (w416:refnum<vi>)
        n189 = control-ref of="Load Parameter"() -> (w413:refnum<vi>)
        n190 = control-ref of="Stop Live"() -> (w411:refnum<vi>)
        n191 = property class="Bool"(reference=w416, "Disabled"=u8 2 ("Deaktiviert")) -> (reference out=w405:refnum<vi>, error out=w404:errorcluster)  [unwired: 1 in]
        n192 = property class="Bool"(reference=w413, "Disabled"=u8 2 ("Deaktiviert")) -> (reference out=w407:refnum<vi>, error out=w406:errorcluster)  [unwired: 1 in]
        n193 = property class="Bool"(reference=w411, "Disabled"=u8 0 ("Deaktiviert")) -> (reference out=w409:refnum<vi>, error out=w408:errorcluster)  [unwired: 1 in]
        n194 = Close Reference(reference=w407, error in (no error)=w406) -> ()  [unwired: 1 out]
        n195 = Close Reference(reference=w405, error in (no error)=w404) -> ()  [unwired: 1 out]
        n196 = Close Reference(reference=w409, error in (no error)=w408) -> ()  [unwired: 1 out]
        n197 = property class="Camera"(reference=w420, error in=w421) -> (error out=w430:errorcluster, "Acquisition"=w429:refnum<k24>)  [unwired: 1 out]
        n198 = invoke class="Acquisition" method="HasStarted"(reference=w429, error in=w430) -> (reference out=w425:refnum<k24>, error out=w424:errorcluster, "HasStarted"=w423:i32, "bValue"=w428:bool)  [unwired: 2 in]
        n199 = invoke class="Acquisition" method="ToString"(reference=w425, error in=w424) -> (error out=w427:errorcluster, "ToString"=w426:string)  [unwired: 1 in, 1 out]
        n200 = call "uc480_Error_Handling.vi"("Error Code"=w423, "Error String"=w426, "Error In"=w427) -> ("Error Out"=w422:errorcluster)  [unwired: 8 in]
        n201 = case shown="False" w428 {
          tunnel: [w433 w443] -> w417
          tunnel: w422 -> [w439 w443]
          tunnel: w420 -> [w438 w442]
          tunnel: [w438 w442] -> w419
          frame False {
            w431 = 1 items=["IS_DONT_WAIT", "IS_WAIT"] ("Wait")
            n202 = property class="Camera"(reference=w438, error in=w439) -> (error out=w440:errorcluster, "Acquisition"=w441:refnum<k24>)  [unwired: 1 out]
            n203 = invoke class="Acquisition" method="Capture"(reference=w441, error in=w440, "param"=w431) -> (reference out=w434:refnum<k24>, error out=w435:errorcluster, "Capture"=w432:i32)  [unwired: 1 in, 1 out]
            n204 = invoke class="Acquisition" method="ToString"(reference=w434, error in=w435) -> (error out=w437:errorcluster, "ToString"=w436:string)  [unwired: 1 in, 1 out]
            n205 = call "uc480_Error_Handling.vi"("Error Code"=w432, "Error String"=w436, "Error In"=w437) -> ("Error Out"=w433:errorcluster)  [unwired: 8 in]
          }
          frame True {
          }
        }
      }
    }
    n206 = call "uc480_SubVI_Example_SyncEventLoop.vi"("Error In"=w36, "use sync"=w38, ".NET (Reference)"=w37) -> ("Error Out"=w34:errorcluster, "Synchronize (ms)"=w35:dbl)  [unwired: 7 in]
    "Error Out" <- w34
    n207 = Wait Until Next ms Multiple(millisecond multiple=w35) -> ()  [unwired: 1 out]
  }
